vi "HEWH Full ERD List.vi"(8 "error in (no error)":errorcluster, 10 "Disable Electronic Mixing Valve (EMV) List":bool, 11 "Disable ERD (Main)":bool) -> (0 "error out":errorcluster, 1 "GEA Inputs":T1 {"Destination" format="%.0x"; "Source" format="%.0x"}, 2 "ERD Headers":string[](array[string]), 3 "Read ERD List":T2[](array[typedef]) {"ERD Number" format="%.0x"})   [LabVIEW 2016]
uses:
  type defs/ERD Read Data In.ctl
  type defs/Data Type.ctl
  type defs/Source_Destination.ctl
  library/GEA2_Toolkit.lvlib
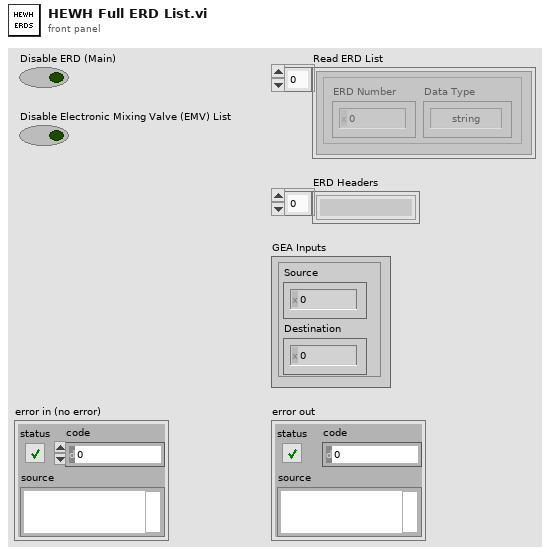
[diagram p1: front panel]
types:
  T1 = typedef "GEA2_Toolkit.lvlib/Source_Destination.ctl" = cluster{"Source":u8, "Destination":u8}
  T2 = typedef "GEA2_Toolkit.lvlib/ERD Read Data In.ctl" = cluster{"ERD Number":u16, "Data Type":T3}
  T3 = typedef "GEA2_Toolkit.lvlib/Data Type.ctl" = enum16{"string", "boolean", "uint8_t", "uint16_t", "uint32_t", "uint64_t"}
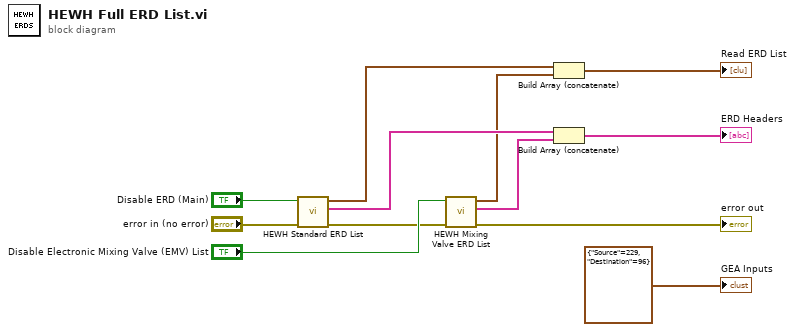
[diagram p0: block diagram]
diagram:
  n1 = call "HEWH Standard ERD List.vi"("Error In"="error in (no error)", "Disable ERD (Main)"="Disable ERD (Main)") -> ("Error Out"=w11:errorcluster, "Header"=w9:string[], "Read ERD List"=w8:T2[])  [unwired: 7 in]
  n2 = call "HEWH Mixing Valve ERD List.vi"("error in (no error)"=w11, "Disable Electronic Mixing Valve (EMV) List"="Disable Electronic Mixing Valve (EMV) List") -> ("error out"=→"error out":errorcluster, "Headers"=w4:string[], "Read ERD List"=w5:T2[])  [unwired: 7 in]
  n3 = Build Array (concatenate)(w8, w5) -> (→"Read ERD List":T2[])
  n4 = Build Array (concatenate)(w9, w4) -> (→"ERD Headers":string[])
  "GEA Inputs" <- T1 {"Source"=229, "Destination"=96} ("GEA Inputs")
